vi "aod_calc_rotate.vi"(8 "FPGA parameters in":T1 {"AOD center frequ. (Hz)_y" format="%.14g"; "AOD half bandwidth_y" format="%.14g"; "AOD Bandwidth_y (Hz)" format="%_6f"; "AOD center frequ. (Hz)_x" format="%.14g"; "cos Phi" format="%.35g"; "sin Phi" format="%.35g"; "AOD_Scale_Factor (1/Zoom)" format="%.35g"; "AOD half bandwidth_x" format="%.14g"; "AOD Bandwidth_x (Hz)" format="%_6f"}, 10 "scaled y input":fxp<+/-,36,32> format="%.14g", 11 "scaled x input":fxp<+/-,36,32> format="%.14g") -> (0 "FPGA parameters out":T1 {"AOD center frequ. (Hz)_y" format="%.14g"; "AOD half bandwidth_y" format="%.14g"; "AOD Bandwidth_y (Hz)" format="%_6f"; "AOD center frequ. (Hz)_x" format="%.14g"; "cos Phi" format="%.35g"; "sin Phi" format="%.35g"; "AOD_Scale_Factor (1/Zoom)" format="%.35g"; "AOD half bandwidth_x" format="%.14g"; "AOD Bandwidth_x (Hz)" format="%_6f"}, 2 "y rotation out":fxp<+/-,36,32> format="%.14g", 3 "x rotation out":fxp<+/-,36,32> format="%.14g")   [LabVIEW 2010]
uses:
  FPGA_parameters_cluster.ctl
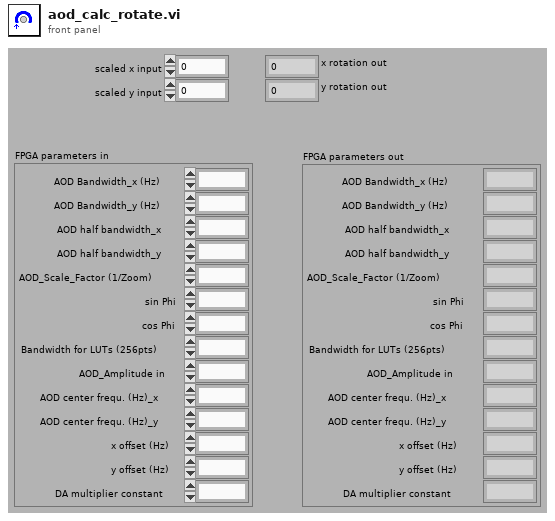
[diagram p1: front panel]
types:
  T1 = typedef "FPGA_parameters_cluster.ctl" = cluster{"AOD Bandwidth_x (Hz)":fxp<+,36,32>, "AOD Bandwidth_y (Hz)":fxp<+,36,32>, "AOD half bandwidth_x":fxp<+,36,32>, "AOD half bandwidth_y":fxp<+,36,32>, "AOD_Scale_Factor (1/Zoom)":fxp<+,36,2>, "sin Phi":fxp<+/-,36,2>, "cos Phi":fxp<+/-,36,2>, "Bandwidth for LUTs (256pts)":fxp<+,36,0>, "AOD_Amplitude in":u16, "AOD center frequ. (Hz)_x":fxp<+,36,32>, "AOD center frequ. (Hz)_y":fxp<+,36,32>, "x offset (Hz)":fxp<+/-,36,32>, "y offset (Hz)":fxp<+/-,36,32>, "DA multiplier constant":fxp<+,64,4>}
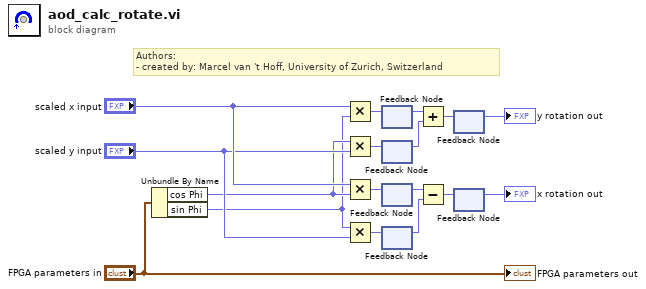
[diagram p0: block diagram]
diagram:
  # "Authors: \n- created by: Marcel van 't Hoff, University of Zurich, Switzerland"
  n1 = Unbundle By Name("FPGA parameters in") -> ("cos Phi"=w3:fxp<+/-,36,2>, "sin Phi"=w2:fxp<+/-,36,2>)
  n2 = Multiply(x="scaled x input", y=w2) -> (x*y=w17:fxp<+/-,36,32>)
  n3 = Multiply(x=w3, y="scaled y input") -> (x*y=w8:fxp<+/-,36,32>)
  n4 = Multiply(x="scaled x input", y=w3) -> (x*y=w13:fxp<+/-,36,32>)
  n5 = Multiply(x=w2, y="scaled y input") -> (x*y=w15:fxp<+/-,36,32>)
  n6 = feedback-in #1(w17) -> ()
  n7 = feedback #1() -> (w16:fxp<+/-,36,32>)  [unwired: 1 out]
  n8 = feedback-in #2(w8) -> ()
  n9 = feedback #2() -> (w6:fxp<+/-,36,32>)  [unwired: 1 out]
  n10 = feedback-in #3(w13) -> ()
  n11 = feedback #3() -> (w10:fxp<+/-,36,32>)  [unwired: 1 out]
  n12 = feedback-in #4(w15) -> ()
  n13 = feedback #4() -> (w9:fxp<+/-,36,32>)  [unwired: 1 out]
  n14 = Add(x=w16, y=w6) -> (x+y=w14:fxp<+/-,36,32>)
  n15 = Subtract(x=w10, y=w9) -> (x-y=w11:fxp<+/-,36,32>)
  n16 = feedback-in #5(w14) -> ()
  n17 = feedback #5() -> (→"y rotation out":fxp<+/-,36,32>)  [unwired: 1 out]
  n18 = feedback-in #6(w11) -> ()
  n19 = feedback #6() -> (→"x rotation out":fxp<+/-,36,32>)  [unwired: 1 out]
  "FPGA parameters out" <- "FPGA parameters in"
